vi "GOOP_TemplateRename.vi"(7 "Pattern":T1=2 items=["4x4x4", "5x6x5", "6x8x6"], 11 "TemplateIn":string) -> (3 "TemplateOut":string)   [LabVIEW 2020]
uses:
  <resource>/Framework/Providers/Open_GDS/ClassProviders/Common/ScriptingFunctions/Scripting_ConnectorPanePatternType.ctl
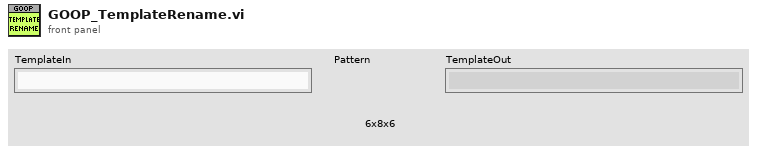
[diagram p1: front panel]
types:
  T1 = typedef "Scripting_ConnectorPanePatternType.ctl" = u16
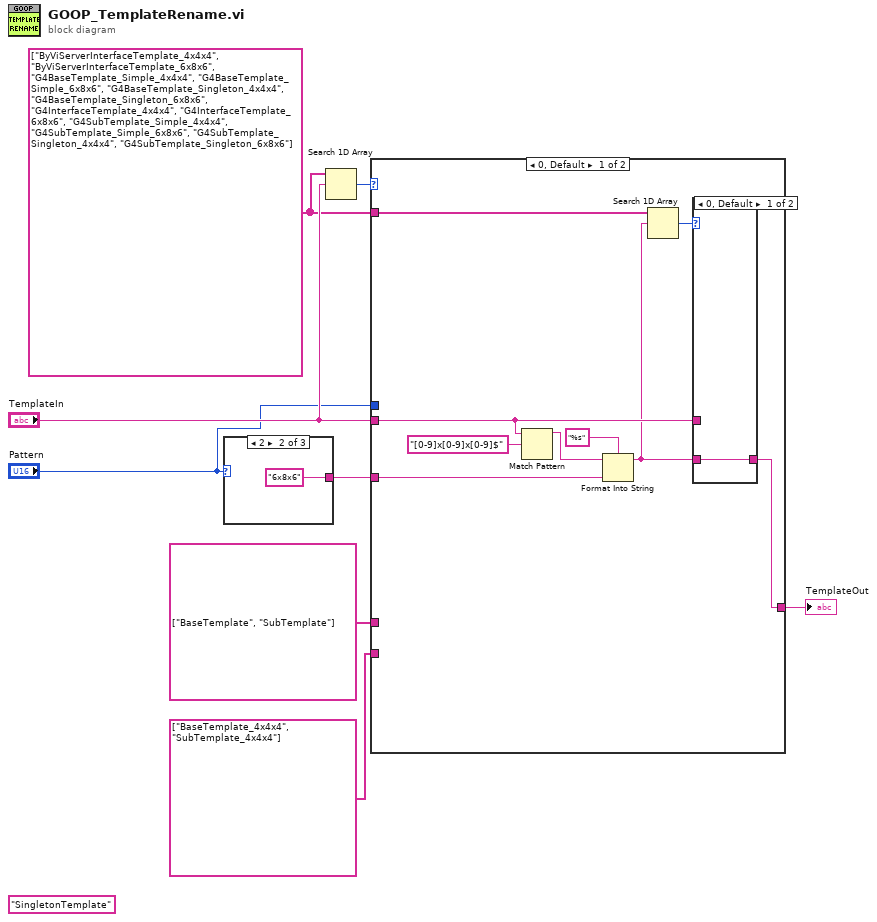
[diagram p0: block diagram]
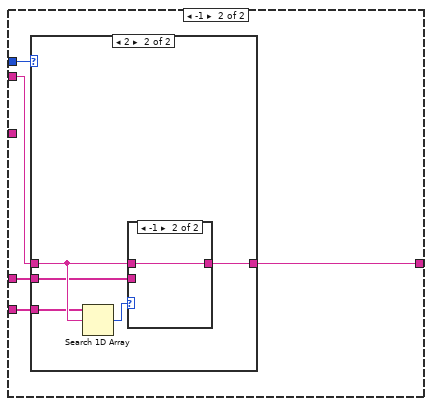
[diagram p3: hidden frame]
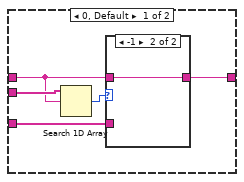
[diagram p4: hidden frame]
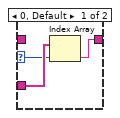
[diagram p5: hidden frame]
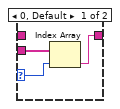
[diagram p6: hidden frame]
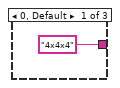
[diagram p7: hidden frame]
diagram:
  (unwired) "SingletonTemplate" ("name")
  w6 = string[] ["ByViServerInterfaceTemplate_4x4x4", "ByViServerInterfaceTemplate_6x8x6", "G4BaseTemplate_Simple_4x4x4", "G4BaseTemplate_Simple_6x8x6", "G4BaseTemplate_Singleton_4x4x4", "G4BaseTemplate_Singleton_6x8x6", "G4InterfaceTemplate_4x4x4", "G4InterfaceTemplate_6x8x6", "G4SubTemplate_Simple_4x4x4", "G4SubTemplate_Simple_6x8x6", "G4SubTemplate_Singleton_4x4x4", "G4SubTemplate_Singleton_6x8x6"] ("Array")
  n1 = case shown="2" "Pattern" {
    tunnel: ["4x4x4" ("name") "6x8x6" ("name") _] -> w7
    frame 0, Default {
    }
    frame 2 {
    }
    frame 1 {
    }
  }
  n2 = Search 1D Array(1D array=w6, element="TemplateIn") -> (index of element=w5:i32)  [unwired: 1 in]
  n3 = case shown="0, Default" w5 {
    tunnel: "TemplateIn" -> [w13 w25]
    tunnel: w7 -> [w16 _]
    tunnel: w6 -> [w15 _]
    tunnel: [w12 w22] -> w4
    tunnel: "Pattern" -> [_ w26]
    tunnel: string[] ["BaseTemplate", "SubTemplate"] -> [_ w24]
    tunnel: string[] ["BaseTemplate_4x4x4", "SubTemplate_4x4x4"] -> [_ w23]
    frame 0, Default {
      n4 = Match Pattern(string=w13, regular expression="[0-9]x[0-9]x[0-9]$") -> (before substring=w18:string)  [unwired: 1 in, 3 out]
      n5 = Format Into String(format string="%s", initial string=w18, w16) -> (resulting string=w11:string)  [unwired: 1 in, 1 out]
      n6 = Search 1D Array(1D array=w15, element=w11) -> (index of element=w14:i32)  [unwired: 1 in]
      n7 = case shown="0, Default" w14 {
        tunnel: w13 -> [_ w21]
        tunnel: [w20 w21] -> w12
        tunnel: w11 -> [w20 _]
        frame 0, Default {
        }
        frame -1 {
        }
      }
    }
    frame -1 {
      n8 = case shown="2" w26 {
        tunnel: w25 -> [w27 w38]
        tunnel: w24 -> [w31 w36]
        tunnel: w23 -> [w29 w37]
        tunnel: [w28 w39] -> w22
        frame 0, Default {
          n9 = Search 1D Array(1D array=w31, element=w27) -> (index of element=w30:i32)  [unwired: 1 in]
          n10 = case shown="-1" w30 {
            selector: w30 -> [w33 _]
            tunnel: w29 -> [w34 _]
            tunnel: [w32 w35] -> w28
            tunnel: w27 -> [_ w35]
            frame 0, Default {
              n11 = Index Array(array=w34, index=w33) -> (element=w32:string)
            }
            frame -1 {
            }
          }
        }
        frame 2 {
          n12 = Search 1D Array(1D array=w37, element=w38) -> (index of element=w40:i32)  [unwired: 1 in]
          n13 = case shown="-1" w40 {
            selector: w40 -> [w42 _]
            tunnel: w36 -> [w43 _]
            tunnel: [w41 w44] -> w39
            tunnel: w38 -> [_ w44]
            frame 0, Default {
              n14 = Index Array(array=w43, index=w42) -> (element=w41:string)
            }
            frame -1 {
            }
          }
        }
      }
    }
  }
  "TemplateOut" <- w4
